vi "StaticVI_reference.vi"() -> ()   [LabVIEW 2017]
panel:
  out "error out":errorcluster
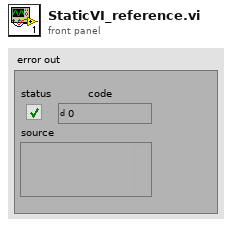
[diagram p1: front panel]
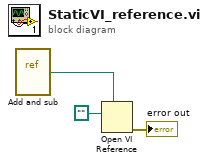
[diagram p0: block diagram]
diagram:
  n1 = vi-ref "Add and sub.vi"() -> (w1:refnum<vi>)
  n2 = Open VI Reference(type specifier VI Refnum (for type only)=w1, vi path=path "") -> (error out=→"error out":errorcluster)  [unwired: 4 in, 1 out]
